vi "positionLogSaver.vi"(10 "Stage position":T1, 11 "file path (use dialog)":path) -> ()   [LabVIEW 2020]
uses:
  typedefs/typedef_stage_position.ctl
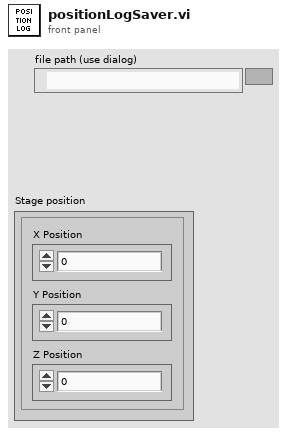
[diagram p1: front panel]
types:
  T1 = typedef "typedef_stage_position.ctl" = cluster{"X Position":dbl, "Y Position":dbl, "Z Position":dbl}
  T2 = enum16{"open", "replace", "create", "open or create", "replace or create", "replace or create with confirmation"}
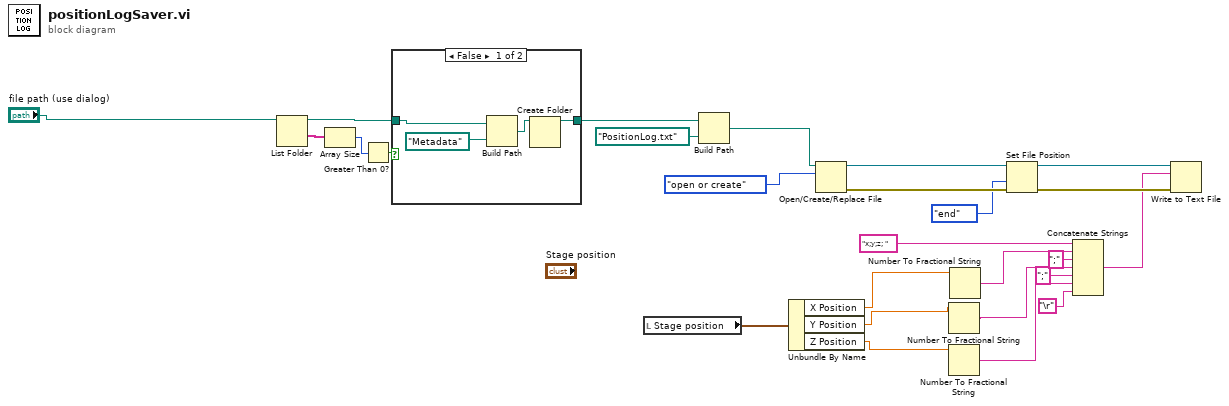
[diagram p0: block diagram]
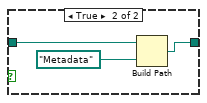
[diagram p2: hidden frame]
diagram:
  n1 = List Folder(path="file path (use dialog)") -> (path out=w2:path, folder names=w6:string[])  [unwired: 3 in, 2 out]
  n2 = Array Size(array=w6) -> (size(s)=w4:i32)
  n3 = Greater Than 0?(x=w4) -> (x > 0?=w5:bool)
  n4 = case shown="False" w5 {
    tunnel: [w30 w31] -> w3
    tunnel: w2 -> [w28 w32]
    frame False {
      n5 = Build Path(base path=w28, name or relative path=path "Metadata") -> (appended path=w27:path)
      n6 = Create Folder(path (use dialog)=w27) -> (created path=w30:path)  [unwired: 2 in, 2 out]
    }
    frame True {
      n7 = Build Path(base path=w32, name or relative path=path "Metadata") -> (appended path=w31:path)
    }
  }
  n8 = local read "Stage position"() -> (w14:T1)
  n9 = Build Path(base path=w3, name or relative path=path "PositionLog.txt") -> (appended path=w7:path)
  n10 = Unbundle By Name(w14) -> ("X Position"=w15:dbl, "Y Position"=w11:dbl, "Z Position"=w9:dbl)
  n11 = Open/Create/Replace File(file path (use dialog)=w7, operation (0:open)=T2."open or create") -> (refnum out=w26:refnum<file>, error out=w25:errorcluster)  [unwired: 4 in, 1 out]
  n12 = Number To Fractional String(number=w11) -> (F-format string=w12:string)  [unwired: 3 in]
  n13 = Number To Fractional String(number=w9) -> (F-format string=w10:string)  [unwired: 3 in]
  n14 = Number To Fractional String(number=w15) -> (F-format string=w20:string)  [unwired: 3 in]
  n15 = Set File Position(refnum=w26, from (0:start)=enum16{"start", "end", "current"}."end", error in=w25) -> (refnum out=w23:refnum<file>, error out=w22:errorcluster)  [unwired: 1 in]
  n16 = Concatenate Strings("x;y;z; " ("text"), w20, ";" ("string"), w12, ";" ("string"), w10, "\r") -> (w19:string)
  n17 = Write to Text File(file (use dialog)=w23, text=w19, error in=w22) -> ()  [unwired: 1 in, 3 out]
